vi "BRig_dataTrial_DAB_iSelect_LowProb.vi"() -> (2 "output_DAB_iSelect_LowProb":i32)   [LabVIEW 2014]
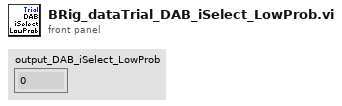
[diagram p1: front panel]
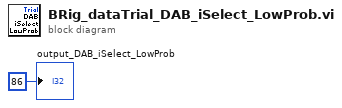
[diagram p0: block diagram]
diagram:
  "output_DAB_iSelect_LowProb" <- 86 ("output_iBlock")
